vi "Viewey Vision Example.vi"() -> ()   [LabVIEW 2015]
panel:
  in  "Input":bool
  in  "Threshold":sgl(knob)=100.0 scale=0.0..200.0
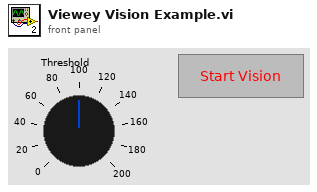
[diagram p1: front panel]
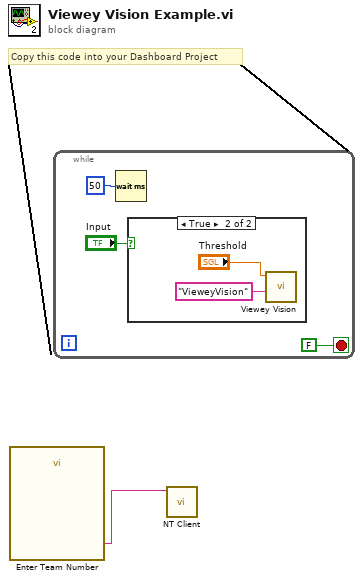
[diagram p0: block diagram]
diagram:
  # "Copy this code into your Dashboard Project"
  n1 = call "Enter Team Number"() -> ("Team Number"=w1:string)  [unwired: 17 in, 2 out]
  n2 = while {
    stop <- FALSE stop-if-true
    n3 = Wait (ms)(milliseconds to wait=u32 50) -> ()  [unwired: 1 out]
    n4 = case shown="True" "Input" {
      frame False {
      }
      frame True {
        n5 = call <userlib>:"Viewey Vision.vi"("Smart Dashboard Name"="VieweyVision", "Threshold"="Threshold") -> ()  [unwired: 10 in]
      }
    }
  }
  n6 = call <vilib>:"NT Client.vi"("Server IP Address"=w1) -> ()  [unwired: 11 in]
